vi "Bind To Name.vi"(8 "error in (no error)":errorcluster, 10 "Type":refnum<class>, 11 "Error Serialization Binder in":refnum<class "Error Serialization Binder.lvclass">) -> (0 "error out":errorcluster, 2 "Type Name":string, 3 "Error Serialization Binder out":refnum<class "Error Serialization Binder.lvclass">)   [LabVIEW 2017, in "Tests.lvlib" / "Error Serialization Binder.lvclass"]
doc: "Controls the binding of a type to a serialized object."
uses:
  Error Serialization Binder.lvclass
  <vilib>/Utility/error.llb/Error Cluster From Error Code.vi
  <vilib>/ErrorRing/Error Ring.xnode
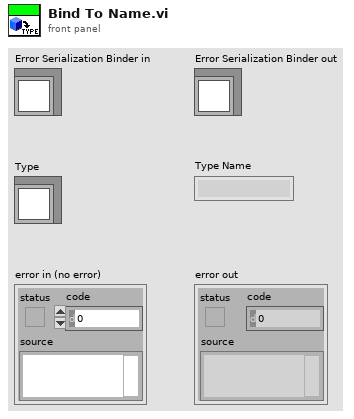
[diagram p1: front panel]
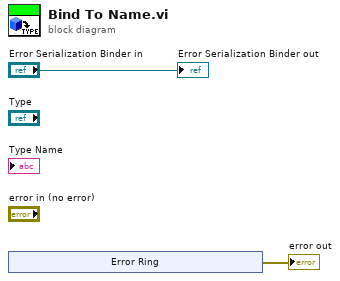
[diagram p0: block diagram]
diagram:
  n1 = xnode "Error Ring"() -> ("error out"=→"error out":errorcluster)
  "Error Serialization Binder out" <- "Error Serialization Binder in"
